vi "RPLiDAR_축변환.vi"(8 "Distance(mm)":dbl[](array[numeric]), 11 "Theta(deg)":dbl[](array[numeric])) -> (0 "Y":dbl[](array[numeric]), 3 "X":dbl[](array[numeric]))   [LabVIEW 2023]
uses:
  <vilib>/Analysis/coordinate.llb/2D Cartesian Coordinate Rotation (Array).vi
  <vilib>/Analysis/NI_AALPro.lvlib
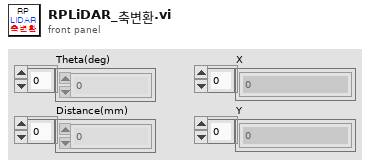
[diagram p1: front panel]
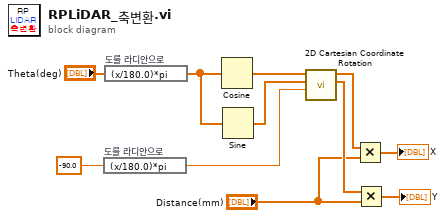
[diagram p0: block diagram]
diagram:
  n1 = expression code="(x/180.0)*pi" "도를 라디안으로"(-90.0 ("theta")) -> (w1:dbl)
  n2 = expression code="(x/180.0)*pi" "도를 라디안으로"("Theta(deg)") -> (w11:dbl[])
  n3 = Cosine(x=w11) -> (cos(x)=w10:dbl[])
  n4 = Sine(x=w11) -> (sin(x)=w9:dbl[])
  n5 = call-poly <vilib>:"2D Cartesian Coordinate Rotation.vi"("theta"=w1, "Y"=w9, "X"=w10) -> ("Y Out"=w6:dbl[], "X Out"=w7:dbl[])  [unwired: 6 in, 1 out]
  n6 = Multiply(x=w7, y="Distance(mm)") -> (x*y=→"X":dbl[])
  n7 = Multiply(x=w6, y="Distance(mm)") -> (x*y=→"Y":dbl[])
